vi "Check_Start_End.vi"(0 "Input Sequence":cluster{string, string[], dbl[], dbl}[](array[cluster])) -> (1 "Syntax Error":bool, 2 "Error Index":i32)   [LabVIEW 2011]
doc: "This VI checks to ensure that every API command in the sequence with an API_Start argument has a corresponding API command with an API_End argument."
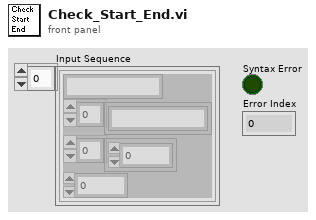
[diagram p1: front panel]
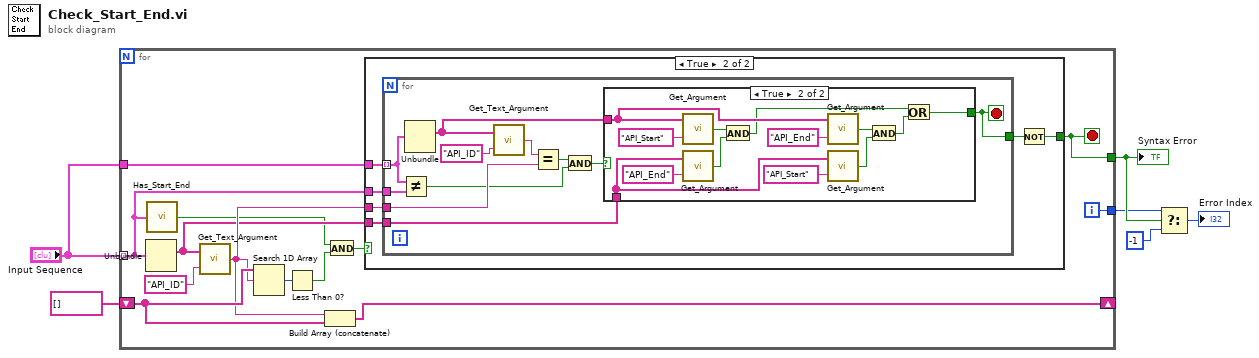
[diagram p0: block diagram]
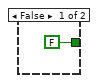
[diagram p2: hidden frame]
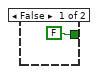
[diagram p3: hidden frame]
diagram:
  n1 = for {
    tunnel: "Input Sequence" -> [w8] mode=indexing
    shift-right: [w18] -> _
    shift-left: string[] [] -> [w14]
    tunnel: "Input Sequence" -> [w17]
    tunnel: [w16] -> w4
    tunnel: [w15] -> w2
    i -> [w15]
    stop <- w16 stop-if-true
    n2 = Unbundle(w8) -> (w11:string[])  [unwired: 3 out]
    n3 = call "Has_Start_End.vi"("Command"=w8) -> ("Has Start and End"=w7:bool)
    n4 = call "Get_Text_Argument.vi"("Argument"="API_ID", "Argument List"=w11) -> ("Text"=w13:string)
    n5 = Search 1D Array(1D array=w14, element=w13) -> (index of element=w12:i32)  [unwired: 1 in]
    n6 = Less Than 0?(x=w12) -> (x < 0?=w9:bool)
    n7 = Build Array (concatenate)(w13, w14) -> (w18:string[])
    n8 = And(x=w7, y=w9) -> (x .and. y?=w10:bool)
    n9 = case shown="True" w10 {
      tunnel: w17 -> [_ w26]
      tunnel: w8 -> [_ w25]
      tunnel: w13 -> [_ w24]
      tunnel: w11 -> [_ w23]
      tunnel: [FALSE w22] -> w16
      frame False {
      }
      frame True {
        n10 = for {
          tunnel: w26 -> [w36] mode=indexing
          tunnel: w25 -> [w37]
          tunnel: w24 -> [w33]
          tunnel: w23 -> [w29]
          tunnel: [w27] -> w21
          stop <- w27 stop-if-true
          n11 = Not Equal?(x=w36, y=w37) -> (x != y?=w31:bool)
          n12 = Unbundle(w36) -> (w30:string[])  [unwired: 3 out]
          n13 = call "Get_Text_Argument.vi"("Argument"="API_ID", "Argument List"=w30) -> ("Text"=w34:string)
          n14 = Equal?(x=w34, y=w33) -> (x = y?=w32:bool)
          n15 = And(x=w32, y=w31) -> (x .and. y?=w28:bool)
          n16 = case shown="True" w28 {
            tunnel: w30 -> [_ w45]
            tunnel: w29 -> [_ w44]
            tunnel: [FALSE w39] -> w27
            frame False {
            }
            frame True {
              n17 = call "Get_Argument.vi"("Argument"="API_Start", "Argument List"=w45) -> ("Enabled"=w49:bool)
              n18 = call "Get_Argument.vi"("Argument"="API_End", "Argument List"=w44) -> ("Enabled"=w48:bool)
              n19 = And(x=w49, y=w48) -> (x .and. y?=w40:bool)
              n20 = call "Get_Argument.vi"("Argument"="API_End", "Argument List"=w45) -> ("Enabled"=w43:bool)
              n21 = call "Get_Argument.vi"("Argument"="API_Start", "Argument List"=w44) -> ("Enabled"=w42:bool)
              n22 = And(x=w43, y=w42) -> (x .and. y?=w41:bool)
              n23 = Or(x=w40, y=w41) -> (x .or. y?=w39:bool)
            }
          }
        }
        n24 = Not(x=w21) -> (.not. x?=w22:bool)
      }
    }
  }
  "Syntax Error" <- w4
  n25 = Select(t=w2, s=w4, f=-1) -> (s? t:f=→"Error Index":i32)
